vi "Processor Assignment Display.vi"(11 "Data Access:Processor":i32) -> (2 "Enabled?":T2(ring), 3 "Mode":T1)   [LabVIEW 2013, in "Standard Engine Editor Node.lvclass"]
uses:
  Standard Engine Editor Node.lvclass
  Processor Assignment Mode.ctl
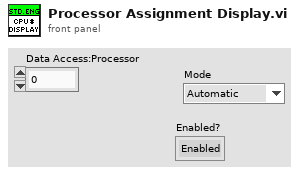
[diagram p1: front panel]
types:
  T1 = typedef "Standard Engine Editor Node.lvclass/Processor Assignment Mode.ctl" = enum16{"Automatic", "Manual"}
  T2 = enum8{"Enabled", "Disabled", "Disabled and Grayed Out"}
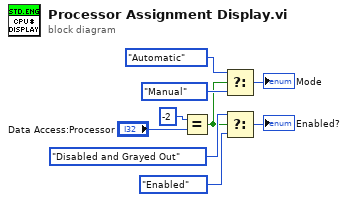
[diagram p0: block diagram]
diagram:
  n1 = Equal?(x=-2, y="Data Access:Processor") -> (x = y?=w3:bool)
  n2 = Select(t=Processor_Assignment_Mode."Automatic" ("Mode"), s=w3, f=Processor_Assignment_Mode."Manual" ("Mode")) -> (s? t:f=→"Mode":T1)
  n3 = Select(t=T2."Disabled and Grayed Out" ("Disabled"), s=w3, f=T2."Enabled") -> (s? t:f=→"Enabled?":T2)
